vi "DEMO.vi"() -> ()   [LabVIEW 2018]
uses:
  <vilib>/picture/picture.llb/imagedata.ctl
  075af626-cc19-402d-99fb-e83e395f8026.vi
  Program Files (x86)/National Instruments/LabVIEW 2018/examples/Design Patterns/Actor Framework/Classes/Customer/Customer.lvclass
  <vilib>/Utility/NIReport.llb/NI_report.lvclass
  <vilib>/LabVIEW Icon API/lv_icon/Classes/Layer/Layer.lvclass
  <vilib>/LabVIEW Icon API/lv_icon/Classes/Icon/Icon.lvclass
  <vilib>/Utility/NIReport.llb/Report Type.ctl
  Class 1.lvclass
  <vilib>/Utility/NIReport.llb/NI_ReportGenerationCore.lvlib
panel:
  in  "Listbox":i32(listbox)=1
  in  "Error In":errorcluster
  out "new picture 2":picture
  out "new picture":picture
  out "2D Picture":picture
  # "Some Custom PopUp Menu Items"
  # "By Paul Alan Cardinale\nRetired Test Engineer"
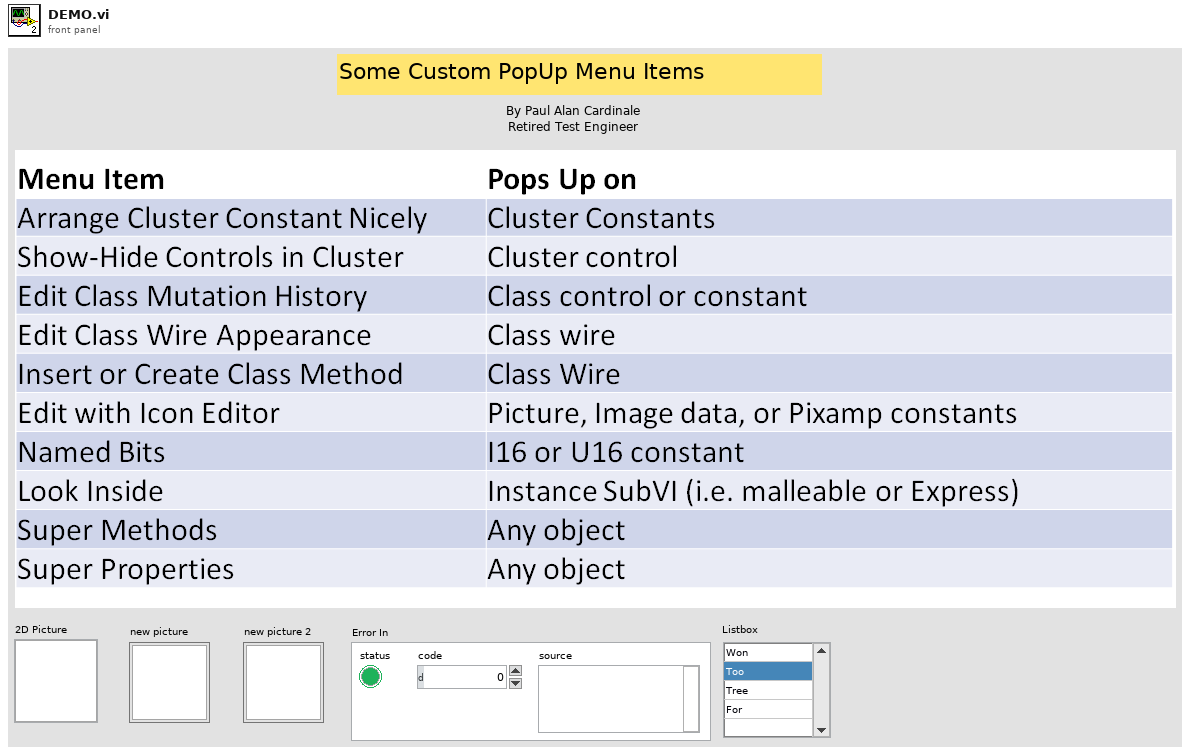
[diagram p1: front panel]
types:
  T1 = enum16{"Arrange Cluster Constants Nicely", "Edit with Icon Editor", "Edit Class Wire Appearance", "Insert or Create Class Method", "Edit Class Mutation History", "Look Inside", "Named Bits", "Show-Hide Controls in Cluster", "Super Methods", "Super Properties"}
  T2 = typedef "NI_ReportGenerationCore.lvlib/Report Type.ctl" = enum16{"HTML", "Word", "Excel"}
  T3 = typedef "imagedata.ctl" = cluster{"image type":i32, "image depth":i32, "image":u8[], "mask":u8[], "colors":u32[], "Rectangle":cluster{"left":i16, "top":i16, "right":i16, "bottom":i16}}
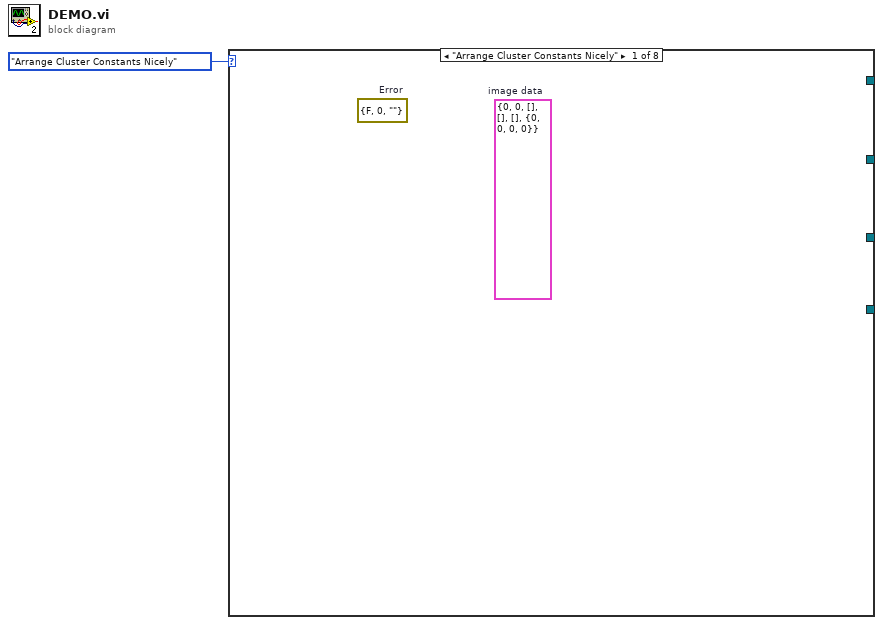
[diagram p0: block diagram]
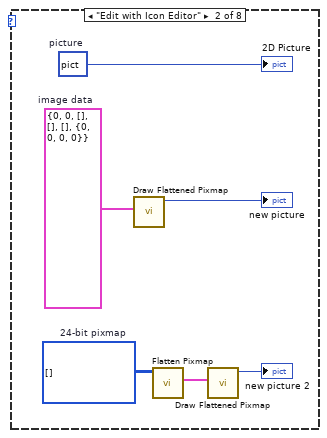
[diagram p2: hidden frame]
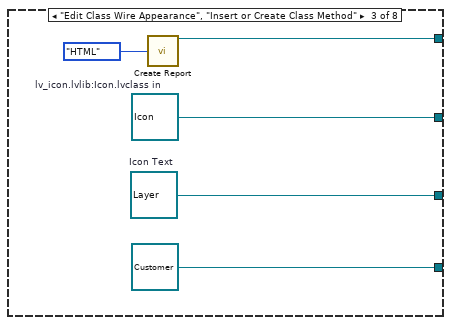
[diagram p3: hidden frame]
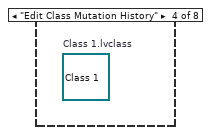
[diagram p4: hidden frame]
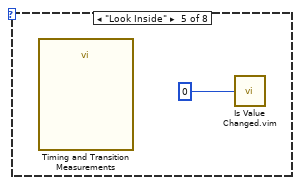
[diagram p5: hidden frame]
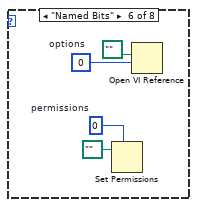
[diagram p6: hidden frame]
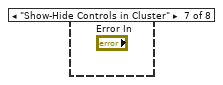
[diagram p7: hidden frame]
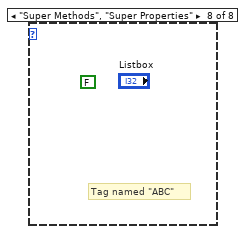
[diagram p8: hidden frame]
diagram:
  n1 = case shown="\"Arrange Cluster Constants Nicely\"" T1."Arrange Cluster Constants Nicely" {
    tunnel: [_ _ w11 _ _ _ _ _] -> _
    tunnel: [_ _ w10 _ _ _ _ _] -> _
    tunnel: [_ _ w9 _ _ _ _ _] -> _
    tunnel: [_ _ refnum<class "Customer.lvclass"> refnum ("Customer.lvlib:Customer.lvclass") _ _ _ _ _] -> _
    frame "Arrange Cluster Constants Nicely" {
      (unwired) T3 {"image type"=0, "image depth"=0, "image"=[], "mask"=[], "colors"=[], "Rectangle"={"left"=0, "top"=0, "right"=0, "bottom"=0}}  # image data
      (unwired) errorcluster {"status"=FALSE, "code"=0, "source"=""}  # Error
    }
    frame "Edit with Icon Editor" {
      w5 = u32[][] []  # 24-bit pixmap
      w2 = picture data[5B]  # picture
      w3 = T3 {"image type"=0, "image depth"=0, "image"=[], "mask"=[], "colors"=[], "Rectangle"={"left"=0, "top"=0, "right"=0, "bottom"=0}}  # image data
      n2 = call <vilib>:"Draw Flattened Pixmap.vi"("image data"=w3) -> ("new picture"=→"new picture":picture)  [unwired: 8 in]
      n3 = call <vilib>:"Flatten Pixmap.vi"("24-bit pixmap"=w5) -> ("image data"=w7:T3)  [unwired: 10 in]
      n4 = call <vilib>:"Draw Flattened Pixmap.vi"("image data"=w7) -> ("new picture"=→"new picture 2":picture)  [unwired: 8 in]
      "2D Picture" <- w2
    }
    frame "Edit Class Wire Appearance", "Insert or Create Class Method" {
      w10 = refnum<class "Layer.lvclass"> refnum  # Icon Text
      w11 = refnum<class "Icon.lvclass"> refnum  # lv_icon.lvlib:Icon.lvclass in
      n5 = call <vilib>:"Create Report.vi"("report type"=Report_Type."HTML") -> ("report out"=w9:refnum<class "NI_report.lvclass">)  [unwired: 13 in, 1 out]
    }
    frame "Edit Class Mutation History" {
      (unwired) refnum<class "Class 1.lvclass"> refnum  # Class 1.lvclass
    }
    frame "Look Inside" {
      n6 = call "Timing and Transition Measurements"() -> ()  [unwired: 11 in, 1 out]
      n7 = call "Is Value Changed.vim"("value"=0) -> ()  [unwired: 1 out]
    }
    frame "Named Bits" {
      w17 = i16 0  # permissions
      w16 = 0  # options
      n8 = Set Permissions(7:w17, 11:path "" ("path")) -> ()  [unwired: 3 in, 2 out]
      n9 = Open VI Reference(vi path=path "", options=w16) -> ()  [unwired: 4 in, 2 out]
    }
    frame "Show-Hide Controls in Cluster" {
    }
    frame "Super Methods", "Super Properties" {
      (unwired) FALSE
      # "Tag named \"ABC\""
    }
  }
